vi "__SISbias_Get.vi"(10 "Bias_LO_equip":T1={"Node address"=19, "CAN Interface"="CAN0", "Cartridge band"=10, "Slave Node in"={"Address"=0, "Serial Number"=[]}, "ObjHandle out"=0, "POL"=1, "sb"=1, "GPIB_SM (SIS S,V)"="24", "GPIB_DMM (SIS I)"="22", "GPIB_SM (MAG I) "="25", "GPIB_SG(LO)"="19", "GPIB_PW (PAMP) "="6", "GPIB_TMP1(8ch)"="12", "GPIB_TMP2(2ch)  "="13", "WCA_avg"=10, "Rsen"=10.0, "BiasModule"=1, "LOModule "=1, "WCA_LO_FREQ_SET"={"YTO Low freq. [GHz]"=14.42, "YTO High freq. [GHz]"=17.7, "Kvco"=1, "Lock Pol."=0, "SET LO FREQ"=72.5, "Multiplier"=6.0, "YTO (HEX)"=0, "YTO coarse( FREQ)"=25.0, "NULL PLL INTEGRATOR"=FALSE}, "Res for"=0} {"Res for" items=["none", "series res", "parallel res"]; "WCA_LO_FREQ_SET"."YTO coarse( FREQ)" min=25 max=150 step=0.0001 format="%.3f"; "WCA_LO_FREQ_SET"."Multiplier" min=3 max=6 step=3; "WCA_LO_FREQ_SET"."SET LO FREQ" min=25 max=150 step=0.0001 format="%.3f"; "WCA_LO_FREQ_SET"."Lock Pol." items=["Lower", "Upper"]; "WCA_LO_FREQ_SET"."Kvco" items=["7.5MHz/V", "15MHz/V"]; "WCA_LO_FREQ_SET"."YTO High freq. [GHz]" format="%.3f"; "WCA_LO_FREQ_SET"."YTO Low freq. [GHz]" format="%.3f"; "LOModule" items=["Manual", "B10Lab LO", "WCA LO"]; "BiasModule" items=["B10Lab Bias", "WCA BiasModule"]; "Slave Node in"."Serial Number" format="%.0x"; "Slave Node in"."Address" format="%.0x"; "Cartridge band" max=10 step=1; "Node address" format="%.0x"}) -> (0 "error out":errorcluster caption="Error out", 1 "Get_I(uA)":dbl, 3 "Get_V(mV)":dbl)   [LabVIEW 2017]
uses:
  <vilib>/express/express arith-compare/Formula/XNode/ExpressFormulaBlockNode.xnode
panel:
  # "LO freq. [GHz]"
  # "YTO LOW\n/High Freq."
  # "ZERO Intgrtr"
  # "Node Address"
  # "Serial Number"
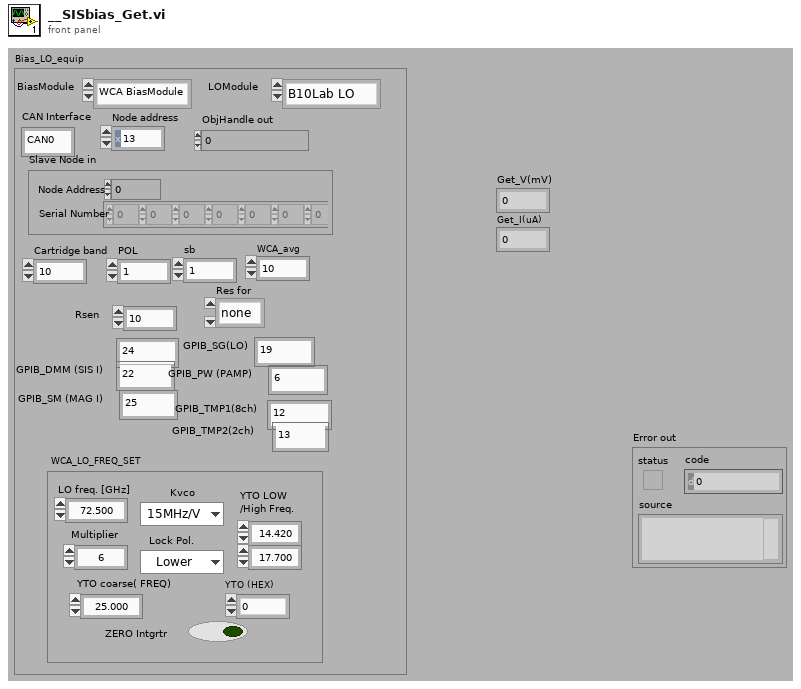
[diagram p1: front panel]
types:
  T1 = cluster{"Node address":u16, "CAN Interface":string, "Cartridge band":u32, "Slave Node in":cluster{"Address":i16, "Serial Number":i8[]}, "ObjHandle out":u32, "POL":u32, "sb":u32, "GPIB_SM (SIS S,V)":string, "GPIB_DMM (SIS I)":string, "GPIB_SM (MAG I) ":string, "GPIB_SG(LO)":string, "GPIB_PW (PAMP) ":string, "GPIB_TMP1(8ch)":string, "GPIB_TMP2(2ch)  ":string, "WCA_avg":i32, "Rsen":dbl, "BiasModule":u16, "LOModule ":u16, "WCA_LO_FREQ_SET":cluster{"YTO Low freq. [GHz]":sgl, "YTO High freq. [GHz]":sgl, "Kvco":u16, "Lock Pol.":u16, "SET LO FREQ":sgl, "Multiplier":sgl, "YTO (HEX)":u16, "YTO coarse( FREQ)":sgl, "NULL PLL INTEGRATOR":bool}, "Res for":u16}
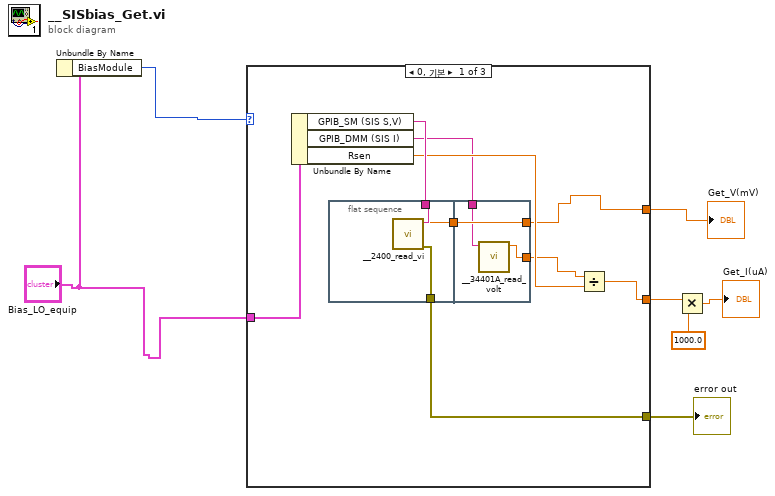
[diagram p0: block diagram]
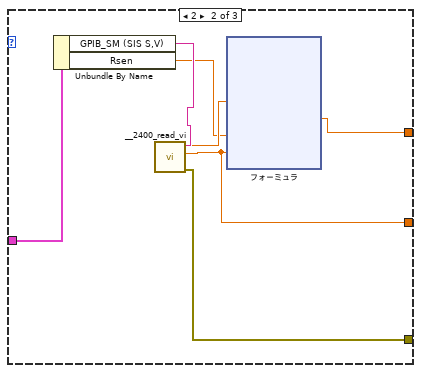
[diagram p2: hidden frame]
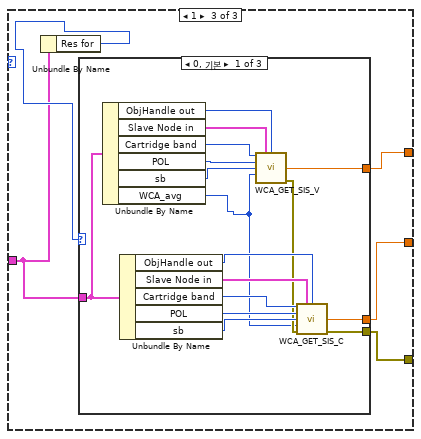
[diagram p3: hidden frame]
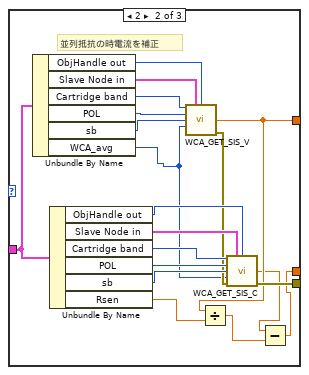
[diagram p4: hidden frame]
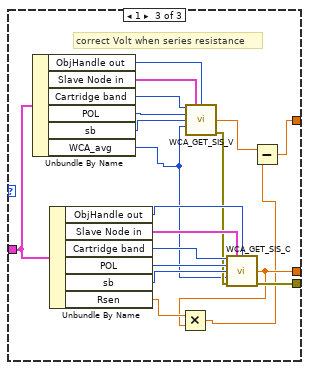
[diagram p5: hidden frame]
diagram:
  n1 = Unbundle By Name("Bias_LO_equip") -> ("BiasModule"=w5:u16)
  n2 = case shown="0, 기본" w5 {
    tunnel: "Bias_LO_equip" -> [w16 w29 w42]
    tunnel: [w11 w24 w45] -> w7
    tunnel: [w12 w23 w46] -> w4
    tunnel: [w13 w27 w44] -> w1
    frame 0, Default {
      n3 = Unbundle By Name(w16) -> ("GPIB_SM (SIS S,V)"=w15:string, "GPIB_DMM (SIS I)"=w9:string, "Rsen"=w14:dbl)
      n4 = flat-sequence {
        tunnel: w15 -> [w19]
        tunnel: [w18] -> w13
        tunnel: [w17] -> w10
        tunnel: [w22] -> w11
        tunnel: w10 -> [w22]
        tunnel: w9 -> [w21]
        tunnel: [w20] -> w8
        frame #0 {
          n5 = call "__2400_read_vi.vi"("GPIB"=w19) -> ("error out"=w18:errorcluster, "volt_read (mV)"=w17:dbl)  [unwired: 4 in, 1 out]
        }
        frame #1 {
          n6 = call "__34401A_read_volt.vi"("GPIB"=w21) -> ("Read_volt(mV)"=w20:dbl)  [unwired: 6 in]
        }
      }
      n7 = Divide(x=w8, y=w14) -> (x/y=w12:dbl)
    }
    frame 2 {
      n8 = Unbundle By Name(w29) -> ("GPIB_SM (SIS S,V)"=w28:string, "Rsen"=w25:dbl)
      n9 = call "__2400_read_vi.vi"("GPIB"=w28) -> ("error out"=w27:errorcluster, "volt_current (mA)"=w23:dbl, "volt_read (mV)"=w26:dbl)  [unwired: 4 in]
      n10 = xnode "フォーミュラ"("v"=w26, "r"=w25, "i"=w23) -> ("結果"=w24:dbl)  [unwired: 1 in, 1 out]
    }
    frame 1 {
      n11 = Unbundle By Name(w42) -> ("Res for"=w43:u16)
      n12 = case shown="0, 기본" w43 {
        tunnel: [w51 w64 w85] -> w46
        tunnel: [w50 w67 w82] -> w45
        tunnel: [w48 w69 w88] -> w44
        tunnel: w42 -> [w47 w68 w87]
        frame 0, Default {
          n13 = Unbundle By Name(w47) -> ("ObjHandle out"=w62:u32, "Slave Node in"=w61:cluster{"Address":i16, "Serial Number":i8[]}, "Cartridge band"=w60:u32, "POL"=w59:u32, "sb"=w58:u32, "WCA_avg"=w49:i32)
          n14 = Unbundle By Name(w47) -> ("ObjHandle out"=w53:u32, "Slave Node in"=w54:cluster{"Address":i16, "Serial Number":i8[]}, "Cartridge band"=w55:u32, "POL"=w56:u32, "sb"=w57:u32)
          n15 = call "WCA_GET_SIS_V.vi"("Cartridge Band"=w60, "Slave Node in"=w61, "ObjHandle in"=w62, "POL"=w59, "sb"=w58, "avg"=w49) -> ("GET_SIS_V"=w50:dbl, "error out"=w52:errorcluster)  [unwired: 7 in, 1 out]
          n16 = call "WCA_GET_SIS_C.vi"("Cartridge Band"=w55, "Slave Node in"=w54, "ObjHandle in"=w53, "POL"=w56, "sb"=w57, "avg"=w49, "error in (no error)"=w52) -> ("GET_SIS_C"=w51:dbl, "error out"=w48:errorcluster)  [unwired: 6 in, 1 out]
        }
        frame 2 {
          # "並列抵抗の時電流を補正"
          n17 = Unbundle By Name(w68) -> ("ObjHandle out"=w81:u32, "Slave Node in"=w80:cluster{"Address":i16, "Serial Number":i8[]}, "Cartridge band"=w79:u32, "POL"=w78:u32, "sb"=w77:u32, "WCA_avg"=w70:i32)
          n18 = Unbundle By Name(w68) -> ("ObjHandle out"=w72:u32, "Slave Node in"=w73:cluster{"Address":i16, "Serial Number":i8[]}, "Cartridge band"=w74:u32, "POL"=w75:u32, "sb"=w76:u32, "Rsen"=w66:dbl)
          n19 = call "WCA_GET_SIS_V.vi"("Cartridge Band"=w79, "Slave Node in"=w80, "ObjHandle in"=w81, "POL"=w78, "sb"=w77, "avg"=w70) -> ("GET_SIS_V"=w67:dbl, "error out"=w71:errorcluster)  [unwired: 7 in, 1 out]
          n20 = Divide(x=w67, y=w66) -> (x/y=w65:dbl)
          n21 = call "WCA_GET_SIS_C.vi"("Cartridge Band"=w74, "Slave Node in"=w73, "ObjHandle in"=w72, "POL"=w75, "sb"=w76, "avg"=w70, "error in (no error)"=w71) -> ("GET_SIS_C"=w63:dbl, "error out"=w69:errorcluster)  [unwired: 6 in, 1 out]
          n22 = Subtract(x=w63, y=w65) -> (x-y=w64:dbl)
        }
        frame 1 {
          # "correct Volt when series resistance"
          n23 = Unbundle By Name(w87) -> ("ObjHandle out"=w100:u32, "Slave Node in"=w99:cluster{"Address":i16, "Serial Number":i8[]}, "Cartridge band"=w98:u32, "POL"=w97:u32, "sb"=w96:u32, "WCA_avg"=w89:i32)
          n24 = Unbundle By Name(w87) -> ("ObjHandle out"=w91:u32, "Slave Node in"=w92:cluster{"Address":i16, "Serial Number":i8[]}, "Cartridge band"=w93:u32, "POL"=w94:u32, "sb"=w95:u32, "Rsen"=w86:dbl)
          n25 = call "WCA_GET_SIS_V.vi"("Cartridge Band"=w98, "Slave Node in"=w99, "ObjHandle in"=w100, "POL"=w97, "sb"=w96, "avg"=w89) -> ("GET_SIS_V"=w84:dbl, "error out"=w90:errorcluster)  [unwired: 7 in, 1 out]
          n26 = call "WCA_GET_SIS_C.vi"("Cartridge Band"=w93, "Slave Node in"=w92, "ObjHandle in"=w91, "POL"=w94, "sb"=w95, "avg"=w89, "error in (no error)"=w90) -> ("GET_SIS_C"=w85:dbl, "error out"=w88:errorcluster)  [unwired: 6 in, 1 out]
          n27 = Multiply(x=w86, y=w85) -> (x*y=w83:dbl)
          n28 = Subtract(x=w84, y=w83) -> (x-y=w82:dbl)
        }
      }
    }
  }
  "Get_V(mV)" <- w7
  "error out" <- w1
  n29 = Multiply(x=w4, y=1000.0) -> (x*y=→"Get_I(uA)":dbl)
